vi "Bitflip Sum.vi"(11 "Proto in":refnum<class "Group.lvclass">) -> (3 "Numeric":u64)   [LabVIEW 2020, in "Group.lvclass"]
uses:
  Group.lvclass
panel:
  out "Reflections":cluster{"Numeric":u64, "Numeric":u64}
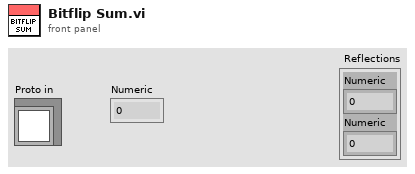
[diagram p1: front panel]
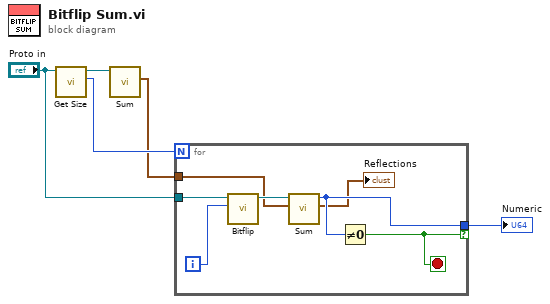
[diagram p0: block diagram]
diagram:
  n1 = call "Get Size.vi"("Proto in"="Proto in") -> ("Size"=w3:i32, "Proto out"=w2:refnum<class "Group.lvclass">)  [unwired: 8 in, 1 out]
  n2 = call "Sum.vi"("Proto In"=w2) -> ("Reflections"=w1:cluster{"Numeric":u64, "Numeric":u64})  [unwired: 9 in, 1 out]
  n3 = for {
    N: w3 -> [_]
    tunnel: "Proto in" -> [w12]
    tunnel: [w8] -> w5 if=w9
    tunnel: w1 -> [w7]
    i -> [w11]
    stop <- w9 stop-if-true
    n4 = call "Bitflip.vi"("index"=w11, "Proto In"=w12) -> ("Proto Out"=w10:refnum<class "Group.lvclass">)  [unwired: 8 in, 1 out]
    n5 = call "Sum.vi"("Reflections to ignore"=w7, "Proto In"=w10) -> ("Reflections"=→"Reflections":cluster{"Numeric":u64, "Numeric":u64}, "Numeric"=w8:u64)  [unwired: 8 in]
    n6 = Not Equal To 0?(x=w8) -> (x != 0?=w9:bool)
  }
  "Numeric" <- w5
